vi "Flush.vi"(8 "error in (no error)":errorcluster, 11 "Sift Client in":refnum<class "Sift Client.lvclass">) -> (0 "error out":errorcluster, 2 "Done":bool, 3 "Sift Client out":refnum<class "Sift Client.lvclass">)   [LabVIEW 2024, in "Sift Client.lvlib" / "Sift Client.lvclass"]
doc: "Flush all samples in the data queue to Sift. This should run in a separate loop from Write. See examples for details."
uses:
  Sift Client.lvclass
  Sift Client.lvclass/Sift Client.ctl
  Sift Client.lvlib
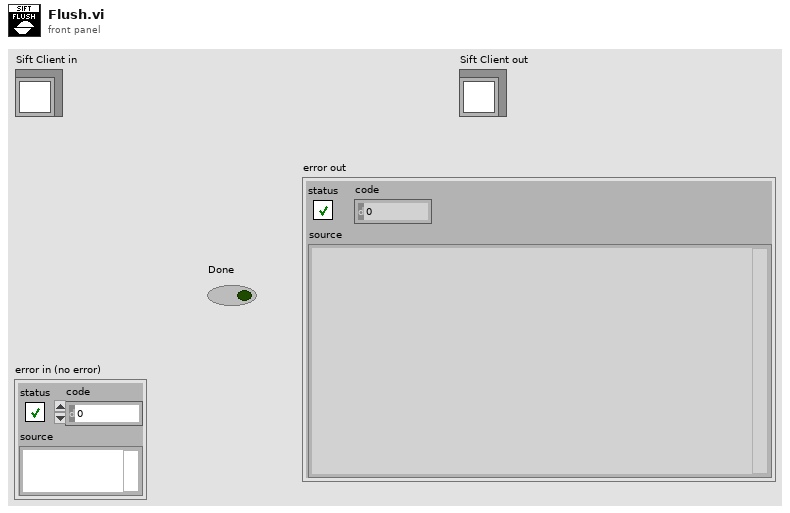
[diagram p1: front panel]
types:
  T1 = typedef "Sift Client.lvlib/Sample.ctl" = cluster{"Flow Name":string, "Timestamp":T2, "Data":string}
  T2 = typedef "Sift Client.lvlib/Timestamp.ctl" = cluster{"seconds":i64, "nanos":i32}
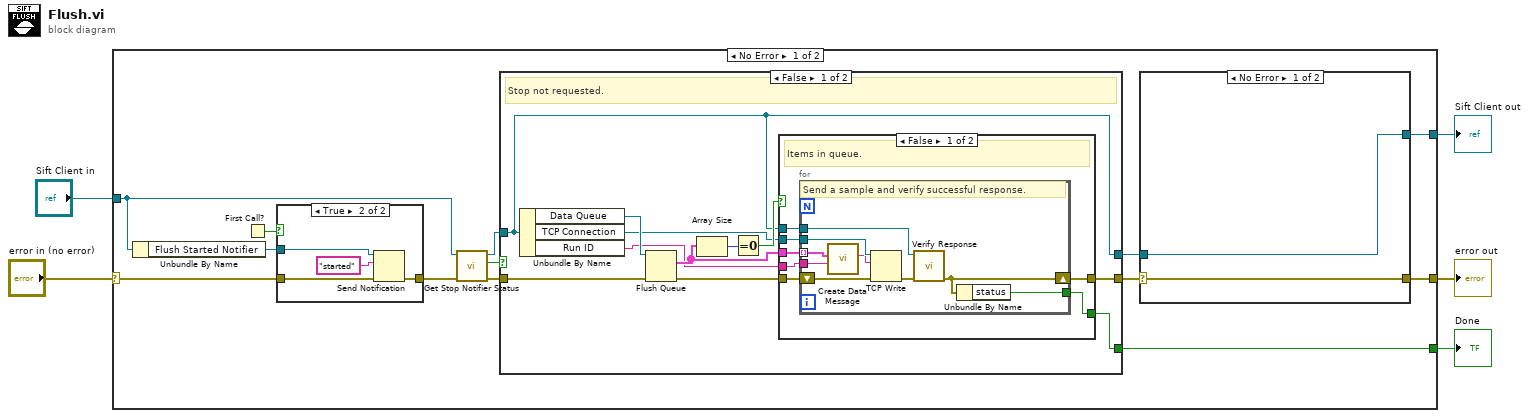
[diagram p0: block diagram]
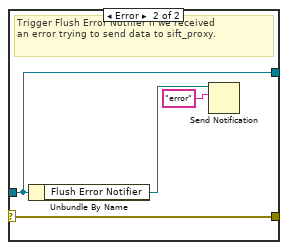
[diagram p3: hidden frame]
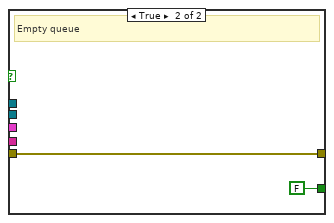
[diagram p4: hidden frame]
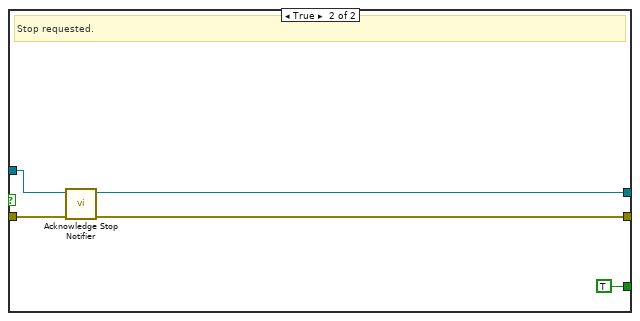
[diagram p5: hidden frame]
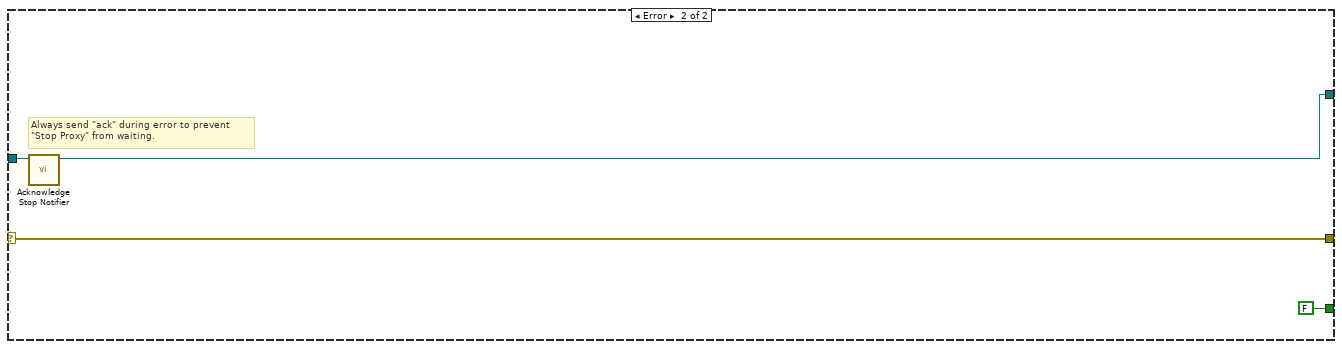
[diagram p6: hidden frame]
diagram:
  n1 = case shown="No Error" "error in (no error)" {
    selector: "error in (no error)" -> [w8 w67]
    tunnel: [w15 w67] -> w4
    tunnel: [w14 w65] -> w2
    tunnel: "Sift Client in" -> [w7 w66]
    tunnel: [w13 FALSE] -> w1
    frame No Error {
      n2 = Unbundle By Name(w7) -> ("Flush Started Notifier"=w12:refnum<notifier>)
      n3 = First Call?() -> (First Call?: T/F=w11:bool)
      n4 = case shown="True" w11 {
        tunnel: w12 -> [_ w23]
        tunnel: [w19 w21] -> w9
        tunnel: w8 -> [w19 w20]
        frame False {
        }
        frame True {
          n5 = Send Notification(notification="started", notifier=w23, error in (no error)=w20) -> (error out=w21:errorcluster)  [unwired: 1 out]
        }
      }
      n6 = call-dynamic "Get Stop Notifier Status.vi"("error in (no error)"=w9, "Sift Client in"=w7) -> ("error out"=w18:errorcluster, "Fired"=w17:bool, "Sift Client out"=w10:refnum<class "Sift Client.lvclass">)  [unwired: 7 in]
      n7 = case shown="False" w17 {
        tunnel: w18 -> [w40 w63]
        tunnel: w10 -> [w30 w61]
        tunnel: [w33 w62] -> w16
        tunnel: [w34 TRUE] -> w13
        tunnel: [w30 w59] -> w6
        frame False {
          # "Stop not requested."
          n8 = Unbundle By Name(w30) -> ("Data Queue"=w39:refnum<queue>, "TCP Connection"=w31:refnum<k5>, "Run ID"=w32:string)
          n9 = Flush Queue(queue=w39, error in (no error)=w40) -> (remaining elements=w36:T1[], error out=w35:errorcluster)  [unwired: 1 out]
          n10 = Array Size(array=w36) -> (size(s)=w38:i32)
          n11 = Equal To 0?(x=w38) -> (x = 0?=w37:bool)
          n12 = case shown="False" w37 {
            tunnel: w36 -> [w47 _]
            tunnel: w31 -> [w46 _]
            tunnel: w32 -> [w45 _]
            tunnel: w35 -> [w43 w58]
            tunnel: [w44 w58] -> w33
            tunnel: [w42 FALSE] -> w34
            tunnel: w30 -> [w41 _]
            frame False {
              # "Items in queue."
              n13 = for {
                tunnel: w47 -> [w56] mode=indexing
                tunnel: w45 -> [w52]
                tunnel: w46 -> [w55]
                shift-right: [w49] -> w44
                shift-left: w43 -> [w54]
                tunnel: [w48] -> w42
                tunnel: w41 -> [w51]
                # "Send a sample and verify successful response."
                n14 = call "Create Data Message.vi"("Run ID"=w52, "Sample"=w56) -> ("Message"=w53:string)  [unwired: 9 in]
                n15 = TCP Write(connection ID=w55, data in=w53, error in (no error)=w54) -> (error out=w50:errorcluster)  [unwired: 1 in, 2 out]
                n16 = call-dynamic "Verify Response.vi"("error in (no error)"=w50, "Sift Client in"=w51) -> ("error out"=w49:errorcluster)  [unwired: 7 in, 2 out]
                n17 = Unbundle By Name(w49) -> ("status"=w48:bool)
              }
            }
            frame True {
              # "Empty queue"
            }
          }
        }
        frame True {
          # "Stop requested."
          n18 = call-dynamic "Acknowledge Stop Notifier.vi"("error in (no error)"=w63, "Sift Client in"=w61) -> ("error out"=w62:errorcluster, "Sift Client out"=w59:refnum<class "Sift Client.lvclass">)  [unwired: 8 in]
        }
      }
      n19 = case shown="No Error" w16 {
        selector: w16 -> [w24 w27]
        tunnel: w6 -> [w25 w26]
        tunnel: [w24 w27] -> w15
        tunnel: [w25 w26] -> w14
        frame No Error {
        }
        frame Error {
          # "Trigger Flush Error Notifier if we received\nan error trying to send data to sift_proxy."
          n20 = Unbundle By Name(w26) -> ("Flush Error Notifier"=w29:refnum<notifier>)
          n21 = Send Notification(notification="error", notifier=w29) -> ()  [unwired: 1 in, 2 out]
        }
      }
    }
    frame Error {
      # "Always send \"ack\" during error to prevent \n\"Stop Proxy\" from waiting."
      n22 = call-dynamic "Acknowledge Stop Notifier.vi"("Sift Client in"=w66) -> ("Sift Client out"=w65:refnum<class "Sift Client.lvclass">)  [unwired: 9 in, 1 out]
    }
  }
  "error out" <- w4
  "Sift Client out" <- w2
  "Done" <- w1
